vi "Set Elevator Position.vi"(8 "error in (no error)":errorcluster, 10 "Elevator Location":T1, 11 "Elevator Controller in":refnum<class "Elevator Controller.lvclass">) -> (0 "error out":errorcluster, 3 "Elevator Controller out":refnum<class "Elevator Controller.lvclass">)   [LabVIEW 2019, in "Elevator Controller.lvlib" / "Elevator Controller.lvclass"]
uses:
  Elevator Controller.lvclass
  Sim Display Console Actor/Elevator Controller/Floors -Enum.ctl
  Elevator Controller.lvclass/Elevator Controller.ctl
  Sim Sensor Interface Actor/Sim Sensor Interface Actor Messages/Write Elevator Position Msg/Write Elevator Position Msg.lvclass/Write Elevator Position Msg.ctl
  <vilib>/ActorFramework/Message Enqueuer/Message Enqueuer.lvclass/Message Enqueuer.ctl
  <vilib>/ActorFramework/Message Enqueuer/Enqueue.vi
  Sim Sensor Interface Actor/Sim Sensor Interface Actor Messages/Write Elevator Position Msg/Write Elevator Position Msg.lvclass
  C:/Program Files (x86)/National Instruments/LabVIEW 2019/vi.lib/ActorFramework/Message/Message.lvclass
  <vilib>/ActorFramework/Message Priority Queue/Priority Enqueue.vi
  Sim Display Console Actor/Elevator Controller/Sim Display Console Actor.lvclass
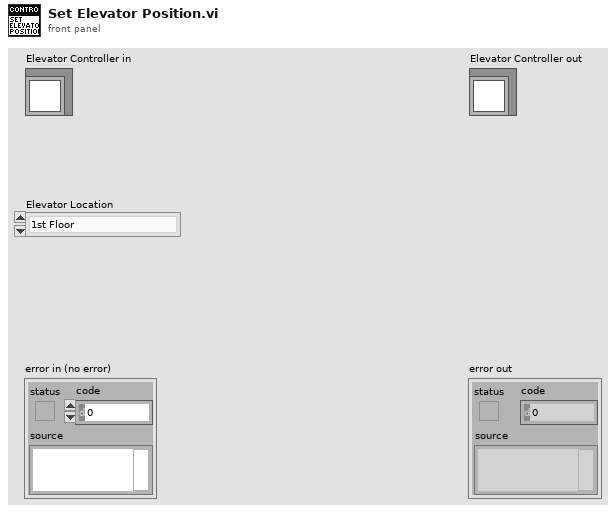
[diagram p1: front panel]
types:
  T1 = typedef "Sim Display Console Actor.lvlib/Sim Display Console Actor.lvclass/Floors -Enum.ctl" = enum16{"1st Floor", "2nd Floor", "3rd Floor", "4th Floor"}
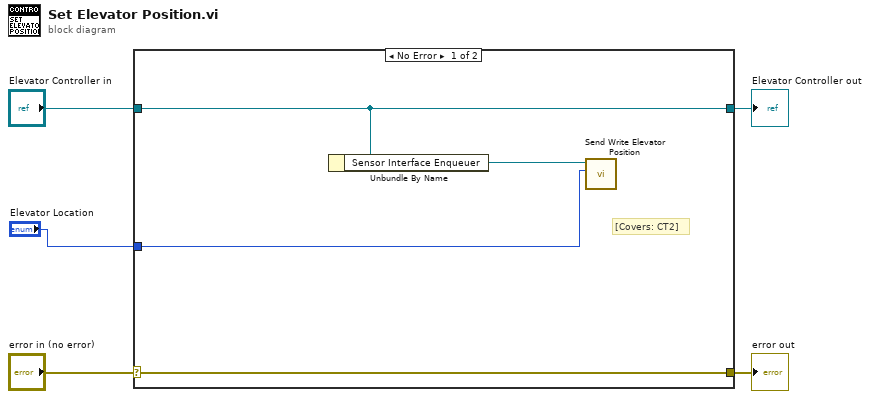
[diagram p0: block diagram]
diagram:
  n1 = case shown="No Error" "error in (no error)" {
    selector: "error in (no error)" -> [w9 w11]
    tunnel: [w9 w11] -> w4
    tunnel: [w8 w10] -> w2
    tunnel: "Elevator Controller in" -> [w8 w10]
    tunnel: "Elevator Location" -> [w6 _]
    frame No Error {
      # "[Covers: CT2]"
      n2 = Unbundle By Name(w8) -> ("Sensor Interface Enqueuer"=w7:refnum<class "Message Enqueuer.lvclass">)
      n3 = call "Send Write Elevator Position.vi"("Elevator Position"=w6, "Message Enqueuer"=w7) -> ()  [unwired: 8 in, 2 out]
    }
    frame Error {
    }
  }
  "error out" <- w4
  "Elevator Controller out" <- w2
